vi "test delta HRT.vi"() -> ()   [LabVIEW 2019]
uses:
  coag.ctl
  model type.ctl
  coag model data.ctl
panel:
  in  "second multiple":sgl
  out "HRT (s)":dbl
  out "total HRT since startup":dbl
  out "sum HRT since dose change":dbl
  out "update coag dose":bool
  in  "data input":T1={"flow rate (L/s)"=0.5, "Raw turbidity (NTU)"=10.0, "floc sed turbidity (NTU)"=0.2}
  in  "Coagulant":T2={"flocculator volume (L)"=1.0, "clarifier volume (L)"=0.5, "dose updates per response delay"=3, "target clarified turbidity (NTU)"=0.3, "Coagulant mode"=enum."simple corrector", "Coag dose [mg/L]"=0.0, "pump mL/rev"=0.0, "clarifier flow [L/s]"=0.5, "min Coag dose [mg/L]"=0.0, "max Coag dose [mg/L]"=0.0, "Steps"=3, "HRT response delay"=2, "kpf"=1.0, "DOM coag demand [mg/L]"=0.0, "min DOM coag demand [mg/L]"=0.0, "max DOM coag demand [mg/L]"=5.0} {"max DOM coag demand [mg/L]" min=0.0 max=20.0 step=0.1; "min DOM coag demand [mg/L]" min=0.0 max=10.0 step=0.1; "DOM coag demand [mg/L]" min=0.0 max=20.0 step=0.1; "HRT response delay" min=1 max=10 step=1; "Steps" min=3 step=1; "clarifier flow [L/s]" min=0.0001 max=1.0 step=0.0001; "target clarified turbidity (NTU)" min=0.1 max=5.0 step=0.01; "dose updates per response delay" min=1 max=100 step=1}
  in  "stop":bool
  out "update DOM demand":bool
  # "ramp controls"
  # "min"
  # "max"
  # "min"
  # "max"
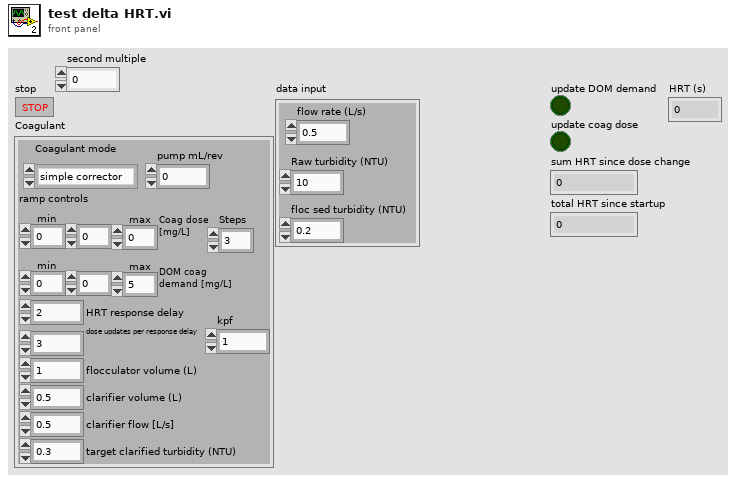
[diagram p1: front panel]
types:
  T1 = typedef "coag model data.ctl" = cluster{"flow rate (L/s)":dbl, "Raw turbidity (NTU)":dbl, "floc sed turbidity (NTU)":dbl}
  T2 = typedef "coag.ctl" = cluster{"flocculator volume (L)":dbl, "clarifier volume (L)":dbl, "dose updates per response delay":u16, "target clarified turbidity (NTU)":dbl, "Coagulant mode":T3, "Coag dose [mg/L]":dbl, "pump mL/rev":dbl, "clarifier flow [L/s]":dbl, "min Coag dose [mg/L]":dbl, "max Coag dose [mg/L]":dbl, "Steps":u16, "HRT response delay":u32, "kpf":dbl, "DOM coag demand [mg/L]":dbl, "min DOM coag demand [mg/L]":dbl, "max DOM coag demand [mg/L]":dbl}
  T3 = typedef "model type.ctl" = enum16{"manual", "ramp", "simple corrector"}
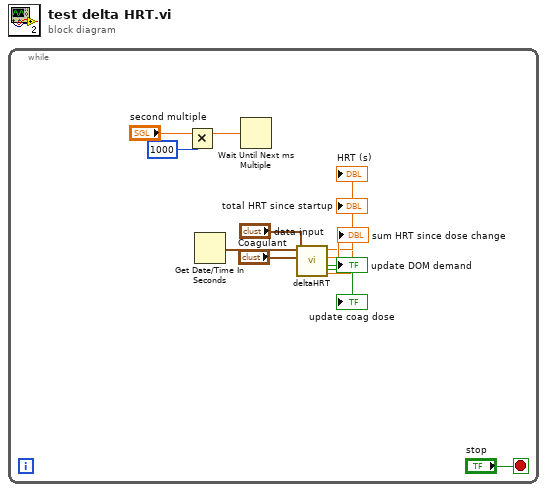
[diagram p0: block diagram]
diagram:
  n1 = while {
    stop <- "stop" stop-if-true
    n2 = Multiply(x="second multiple", y=u32 1000) -> (x*y=w2:sgl)
    n3 = Get Date/Time In Seconds() -> (seconds since 1Jan1904=w12:timestamp)
    n4 = Wait Until Next ms Multiple(millisecond multiple=w2) -> ()  [unwired: 1 out]
    n5 = call "deltaHRT.vi"("data input"="data input", "Coagulant"="Coagulant", "seconds since 1Jan1904"=w12) -> ("HRT (s)"=→"HRT (s)":dbl, "update DOM demand"=→"update DOM demand":bool, "sum HRT since dose change"=→"sum HRT since dose change":dbl, "total HRT since startup"=→"total HRT since startup":dbl, "update coag dose"=→"update coag dose":bool)  [unwired: 4 in]
  }
